vi "Digital_Bridge_3_kart.vi"() -> ()   [LabVIEW 2014] (continued)
                n1468 = call "Kontrol X.vi"("denge degeri"=1.0, "İterasyon Denge"=w4397, "Denge Kosulu x1_x2"=w4399, "Manuel/Otomatik"=w4405, "frekans index"=w4398) -> ("Denge Seçimi"=w4402:u8, "New İterasyon Denge"=w4401:dbl, "Iterasyon Count Successful"=w4400:dbl, "Start Denge X"=w4403:bool)  [unwired: 7 in]
                n1469 = case shown="True" w4403 {
                  tunnel: w4402 -> [w4413 _]
                  tunnel: w4401 -> [_ _]
                  tunnel: w4400 -> [w4412 _]
                  frame False {
                    n1470 = local write "Iterasyon Successful"(w4412) -> ()
                    n1471 = local write "Denge Seçimi"(w4413) -> ()
                    n1472 = local read "iterasyon AD"() -> (w4407:dbl)
                    n1473 = local write "wagner switch"(TRUE ("10R switch")) -> ()
                    n1474 = local write "count meas"(u16 0 ("count meas")) -> ()
                    n1475 = local write "KONTROL X"(FALSE ("KONTROL X")) -> ()
                    n1476 = local write "Boolean"(TRUE ("Boolean 4")) -> ()
                    n1477 = Increment(x=w4407) -> (x+1=w4406:dbl)
                    n1478 = local write "iterasyon AD"(w4406) -> ()
                  }
                  frame True {
                    n1479 = local write "RESET SENS X"(TRUE ("Start Wagner Y")) -> ()
                    n1480 = local write "KONTROL X"(FALSE ("KONTROL X")) -> ()
                  }
                }
              }
            }
            n1481 = case shown="True" "KONTROL Y" {
              frame False {
              }
              frame True {
                n1482 = local read "Outpu Denge Kosulu y1_y2"() -> (w4479:dbl[][])
                n1483 = local read "iterasyon AD"() -> (w4477:dbl)
                n1484 = local read "Manuel/Otomatik"() -> (w4485:enum16{"Manuel", "Otomatik"})
                n1485 = local read "frekans index"() -> (w4478:dbl)
                n1486 = call "Kontrol Y.vi"("denge degeri"=1.0, "İterasyon Denge"=w4477, "Denge Kosulu y1_y2"=w4479, "Manuel/Otomatik"=w4485, "frekans index"=w4478) -> ("Denge Seçimi"=w4482:u8, "New İterasyon Denge"=w4481:dbl, "Iterasyon Count Successful"=w4480:dbl, "Start Denge Y"=w4483:bool)  [unwired: 7 in]
                n1487 = case shown="True" w4483 {
                  tunnel: w4482 -> [w4493 _]
                  tunnel: w4481 -> [_ _]
                  tunnel: w4480 -> [w4492 _]
                  frame False {
                    n1488 = local write "Iterasyon Successful"(w4492) -> ()
                    n1489 = local write "wagner switch"(TRUE ("10R switch")) -> ()
                    n1490 = local write "Denge Seçimi"(w4493) -> ()
                    n1491 = local write "count meas"(u16 0 ("count meas")) -> ()
                    n1492 = local read "iterasyon AD"() -> (w4487:dbl)
                    n1493 = local write "KONTROL Y"(FALSE ("KONTROL Y")) -> ()
                    n1494 = local write "Boolean"(TRUE ("Boolean 4")) -> ()
                    n1495 = Increment(x=w4487) -> (x+1=w4486:dbl)
                    n1496 = local write "iterasyon AD"(w4486) -> ()
                  }
                  frame True {
                    n1497 = local write "RESET SENS Y"(TRUE ("Start Wagner Y")) -> ()
                    n1498 = local write "KONTROL Y"(FALSE ("KONTROL Y")) -> ()
                  }
                }
              }
            }
          }
          frame 2 {
            # "Bu bölümde, ilgili denge durumunun dengede olup olmadığı kontrol edilir.\n\nEğer denge sağlanmışsa, program doğrudan bir sonraki denge aşamasına geçer.\n\nAyrıca, tüm dengeler başarıyla tamamlanmış ve belirlenen ölçüm sayısına ulaşılmışsa, veriler bu alt program (subVI) aracılığıyla Excel dosyasına aktarılır."
            # "Bu bölümde, Y değerinin dengelendiği kabul edilerek, şimdi sıra X değerinin dengede olup olmadığını kontrol etmeye gelir. \n\nEğer X de dengedeyse, program bir sonraki işlem için ilgili switch case’i aktif eder. \n\nAncak Y dengede değilse, program X’i dengelemeye yönelik işlemlere yönlendirilir."
            # "Bu bölümde, X değerinin dengelendiği kabul edilerek, şimdi sıra Y değerinin dengede olup olmadığını kontrol etmeye gelir. \n\nEğer Y de dengedeyse, program bir sonraki işlem için ilgili switch case’i aktif eder. \n\nAncak Y dengede değilse, program Y’yi dengelemeye yönelik işlemlere yönlendirilir."
            # "Bu bölümde ilk olarak giriş (input) değeri sisteme uygulanır. Eğer program ilk kez çalıştırılıyorsa, global input üzerinden belirlenen ilk değer (genellikle 0 V) kullanılır. \n\nArdından, cihazdan X değerleri okunur. Bu işlem 10 kez tekrarlanır ve elde edilen ölçümlerin ortalaması alınarak bir sonuç değeri elde edilir. Bu ortalama değer, daha sonra yapılacak işlemlerde kullanılmak üzere saklanır. Özellikle, formül içinde X değerini sıfırlamak için bu bilgiye ihtiyaç duyulur. \n\nEğer girilen input değeri 8 V’tan büyükse, bu durum sistem için güvenli olmayabileceğinden program hata (error) verir ve işlemi durdurur."
            # "Bu bölümün temel amacı, ölçüm aralığını (range) artırmaktır. Program, cihazdan gelen X ve Y değerlerini okuyarak bu değerlerin belirlenen aralık içinde olup olmadığını kontrol eder. \n\nEğer değerler aralık dışındaysa, aralık tekrar artırılır ve ölçüm yeniden yapılır. \n\nAyrıca, bu süreçte input ve output değerleri global değişkenlere kaydedilir. Çünkü sonraki turda, bu kaydedilen değerler farklı bir ölçüm aralığında eğim hesaplaması için kullanılacaktır."
            # "Bu bölümde, sıfırlanacak değer cihazdan okunur. Eğer okunan değer denge koşulunu sağlıyorsa, program Kontrol Y Case’ine geçer. \n\nAncak denge koşulu sağlanmazsa, program if-else yapısına yönlendirilir ve buna göre işlem devam eder."
            # "Bu bölümde, cihaza ikinci input değeri uygulanır ve karşılık gelen output değeri okunur. Daha sonra, hem input hem de output değerleri bir formüle yerleştirilir. Bu formül sayesinde, cihazın 0’a eşitleyeceği (sıfırlayacağı) yeni bir input değeri hesaplanır ve bu değer cihaza uygulanır."
            # "Auto Phase, Read X1 Y1, Read X2 Y2, Result Phase: \n\nBu bölümler genel olarak faz ölçümü işlemini gerçekleştirir. \n\nİlk olarak, faz değeri 0’a sıfırlanır. Ardından, global input üzerinden belirlenen range (ölçüm aralığı) değeri uygulanır. Bu işlemden sonra yine global input’ta tanımlanmış olan: \n\nInput 1 verilir ve okuma yapılır (Read X1 Y1) \n\nInput 2 verilir ve okuma yapılır (Read X2 Y2) \n\nBu iki ölçüm sonucuna göre faz değeri bir formül yardımıyla hesaplanır. Elde edilen bu yeni faz değeri, ilgili F/P (frekans/faz) dizisine aktarılır. \n\nBu işlemler, sistemin doğru fazla çalışmasını sağlamak ve sonraki işlemlerde bu bilgiyi referans olarak kullanmak için gerçekleştirilir."
            # "X1 2 ile benzer görevi üstleniyor sadece değerler Y oluyor"
            # "IF ELSE X 2 ile benzer görevi üstleniyor sadece değerler Y oluyor"
            # "X 2 ile benzer görevi üstleniyor sadece değerler Y oluyor"
            # "Range Kontrol X 2 ile benzer görevi üstleniyor sadece değerler Y oluyor"
            # "Bu bölümde, daha önce iterasyon (tekrarlama) yapılıp yapılmadığına bakılarak, programın hangi yöne devam edeceğine karar verilir. \n\nEğer gerekli ise, range kontrolü (ölçüm aralığının uygunluğu) yapılır veya sensitivity ayarlama (cihazın duyarlılığını belirleme) bölümlerine yönlendirilir. Bu sayede sistem, ölçüm koşullarına en uygun şekilde ayarlanarak doğru ve güvenilir sonuçlar elde edilmesi sağlanır."
            # "Bu bölümde, daha önce belirlenen F/P dizilerindeki (frekans/faz değerleri) faz bilgileri, mevcut frekansa göre uygulanır. Ardından, ilgili denge koşulunun daha önce gerçekleştirilip gerçekleştirilmediği kontrol edilir. \nEğer bu denge daha önce sağlanmamışsa, program uygun faz ayarlamasını yapar. Ancak denge daha önce zaten kurulmuşsa, faz ayarı yapılmadan işleme devam edilir. Bu sayede gereksiz tekrarların önüne geçilmiş olur."
            # "Bu bölüm, iterasyona (tekrarlamalı işleme) bağlı olarak Reserve ayarının maksimumda mı yoksa minimumda mı olacağını belirler. Aynı zamanda, ölçüm sürecinin başlangıcında kullanılacak olan sensitivity  değerleri de bu bölümde ayarlanır. Bu ayarlar, ölçüm sırasında cihazın hassasiyetini ve çalışma aralığını doğru şekilde belirlemek için gereklidir."
            # "Bu bölümde öncelikle, sistemin kaç kez ölçüm yaptığına işaret eden meas number (ölçüm sayısı) kontrol edilir. \nEğer bu sayı 6’dan büyükse (bu sınır kullanıcı tarafından belirlenmiştir ve değiştirilebilir), program hata verir ve reset values adlı bölüme yönlenir. Bu durum, sistemin çok fazla başarısız deneme yapmasını engellemek içindir. \nEğer ölçüm sayısı 6’dan küçükse, program global bir değişken olan sensitivity (duyarlılık) değerini ayarlar ve ardından işlemlere devam etmek üzere Start X bölümüne geçer."
            # "Bu bölümde, ölçüm için gerekli olan giriş (input) değerleri sisteme girilir. Girişler tamamlandıktan sonra program, ölçüm işlemini başlatmak üzere X adlı bölüme yönlendirilir. Bu adım, ölçüm sürecinin fiilen başlatıldığı ilk noktadır."
            # "Pass subvi girmeden önce doğru range miyiz değil miyiz ölçüyor, değil ise +2 üst kademeye gidiyor"
            # "Start 10R X ile benzer görevi üstleniyor sadece değerler Y oluyor"
            # "Reset Sens X 2 ile benzer görevi üstleniyor sadece değerler Y oluyor"
            # "Start X 2 ile benzer görevi üstleniyor sadece değerler Y oluyor"
            # "10R"
            n1499 = case shown="True" "Start 10R Y" {
              frame False {
              }
              frame True {
                n1500 = flat-sequence {
                  tunnel: [w5317] -> w5305
                  tunnel: [w5316] -> w5304
                  tunnel: w5305 -> [w5321]
                  tunnel: w5304 -> [w5320]
                  frame #0 {
                    n1501 = local read "frekans index"() -> (w5311:dbl)
                    n1502 = local read "Frekanslar"() -> (w5312:dbl[])
                    n1503 = local read "Direnc 1 - Direnc 2"() -> (w5314:u32)
                    n1504 = local read "10R F/P Array"() -> (w5315:dbl[][])
                    n1505 = Index Array(array=w5312, index=w5311) -> (element=w5313:dbl)
                    n1506 = call "get_phase_element.vi"("index r"=w5314, "hz"=w5313, "Array"=w5315) -> ("element"=w5307:dbl)  [unwired: 8 in]
                    n1507 = Number To Fractional String(number=w5307) -> (F-format string=w5308:string)  [unwired: 3 in]
                    n1508 = Search and Replace String(input string=w5308, search string=",", replace string="." ("replace string (\"\")")) -> (result string=w5306:string)  [unwired: 5 in, 3 out]
                    n1509 = local read "GPIB In"() -> (w5318:refnum<visa-resource-name>)
                    n1510 = call "reference phase.vi"("Reference Phase (0.000 degrees)"=w5306, "VISA resource name"=w5318) -> ("error out"=w5316:errorcluster, "VISA resource name out"=w5317:refnum<visa-resource-name>)  [unwired: 8 in]
                  }
                  frame #1 {
                    w5319 = u16 0 items=["A", "A-B"] ("Input Source (0: A)")
                    n1511 = call "input source.vi"("error in (no error)"=w5320, "Input Source (0: A)"=w5319, "VISA resource name"=w5321) -> ()  [unwired: 7 in, 2 out]
                  }
                  frame #2 {
                    n1512 = local write "Boolean 2"(FALSE ("Boolean 4")) -> ()
                    n1513 = local write "RESET SENS Y 2"(TRUE ("START X")) -> ()
                    n1514 = local write "Start 10R Y"(FALSE ("START Y 6")) -> ()
                  }
                }
              }
            }
            n1515 = case shown="True" "10R switch" {
              frame False {
              }
              frame True {
                n1516 = flat-sequence {
                  frame #0 {
                    n1517 = local read "iterasyon 10R"() -> (w5245:dbl)
                    n1518 = Equal?(x=w5245, y=0.0) -> (x = y?=w5246:bool)
                    n1519 = case shown="True" w5246 {
                      frame False {
                      }
                      frame True {
                        n1520 = local read "1 or 10"() -> (w5248:i32)
                        n1521 = case shown="1" w5248 {
                          frame 0, Default {
                          }
                          frame 1 {
                            n1522 = local write "iterasyon 10R"(1.0 ("iterasyon WAGNER")) -> ()
                          }
                        }
                      }
                    }
                  }
                  frame #1 {
                    n1523 = local read "iterasyon 10R"() -> (w5251:dbl)
                    n1524 = Greater?(x=w5251, y=0.0) -> (0:w5250:bool)
                    n1525 = case shown="True" w5250 {
                      frame False {
                        n1526 = local read "Reserve 10R"() -> (w5254:u16)
                        n1527 = case shown="2" w5254 {
                          tunnel: ["0" ("Reserve(MAX-MIN)") "1" ("Reserve(MAX-MIN)") "2" ("Reserve(MAX-MIN)")] -> w5253
                          frame 0, Default {
                          }
                          frame 1 {
                          }
                          frame 2 {
                          }
                        }
                        n1528 = local read "GPIB In"() -> (w5255:refnum<visa-resource-name>)
                        n1529 = call "Reserve.vi"("Reserve(MAX-MIN)"=w5253, "VISA resource name"=w5255) -> ()  [unwired: 8 in, 2 out]
                      }
                      frame True {
                        n1530 = local read "GPIB In"() -> (w5260:refnum<visa-resource-name>)
                        n1531 = call "Reserve.vi"("Reserve(MAX-MIN)"="0", "VISA resource name"=w5260) -> ()  [unwired: 8 in, 2 out]
                      }
                    }
                  }
                  frame #2 {
                    n1532 = Wait (ms)(milliseconds to wait=u32 500) -> ()  [unwired: 1 out]
                  }
                  frame #3 {
                    w5263 = u16 1 items=["Wagner", "Ground"] ("Switch")
                    w5264 = u16 2 items=["Open All", "Ana Denge", "10R", "1R"] ("Ring")
                    n1533 = call "mux1.vi"("Ring"=w5264) -> ("error out"=w5265:errorcluster)  [unwired: 9 in]
                    n1534 = property on="Tab Control" class="TabCtl (strict)"("Value"=T4."10R" ("Tab Control")) -> ()  [unwired: 2 in, 2 out]
                    n1535 = call "mux2.vi"("Switch"=w5263, "error in (no error)"=w5265) -> ()  [unwired: 6 in, 1 out]
                  }
                  frame #4 {
                    n1536 = Wait (ms)(milliseconds to wait=u32 1000) -> ()  [unwired: 1 out]
                  }
                  frame #5 {
                    n1537 = local read "1 or 10"() -> (w5270:i32)
                    n1538 = local read "İterasyon X 2"() -> (w5273:dbl)
                    n1539 = Equal?(x=w5270, y=1) -> (x = y?=w5269:bool)
                    n1540 = Greater?(x=w5273, y=0.0) -> (0:w5268:bool)
                    n1541 = Or(x=w5268, y=w5269) -> (x .or. y?=w5267:bool)
                    n1542 = case shown="False" w5267 {
                      frame False {
                        n1543 = local read "X Range 10R"() -> (w5275:dbl)
                        n1544 = local read "Y Range 10R"() -> (w5274:dbl)
                        n1545 = global write "show_sensitivity.vi" "show sensitivity (10R  x)"(w5275) -> ()
                        n1546 = global write "show_sensitivity.vi" "show sensitivity (10R  y)"(w5274) -> ()
                      }
                      frame True {
                        w5276 = 16.0 ("Max. Hassasiyet")
                        n1547 = global write "show_sensitivity.vi" "show sensitivity (10R  x)"(w5276) -> ()
                        n1548 = global write "show_sensitivity.vi" "show sensitivity (10R  y)"(w5276) -> ()
                      }
                    }
                  }
                  frame #6 {
                    n1549 = local write "Start 10R X"(TRUE ("START WAGNER")) -> ()
                    n1550 = local write "10R switch"(FALSE ("wagner switch")) -> ()
                  }
                }
              }
            }
            n1551 = case shown="True" "RESET SENS Y 2" {
              frame False {
              }
              frame True {
                n1552 = local read "count meas"() -> (w5284:u16)
                n1553 = local read "iterasyon 10R"() -> (w5282:dbl)
                n1554 = Greater?(x=w5284, y=u16 8) -> (0:w5281:bool)
                n1555 = Greater?(x=w5282, y=10.0) -> (0:w5280:bool)
                n1556 = Or(x=w5281, y=w5280) -> (x .or. y?=w5279:bool)
                n1557 = case shown="True" w5279 {
                  frame False {
                    n1558 = flat-sequence {
                      frame #0 {
                        n1559 = global read "show_sensitivity.vi" "show sensitivity (10R  y)"() -> (w5286:dbl)
                        n1560 = local read "GPIB In"() -> (w5287:refnum<visa-resource-name>)
                        n1561 = call "get_sensitivity.vi"("input 1"=w5286, "SR850 GPIB In"=w5287) -> ()  [unwired: 8 in, 2 out]
                      }
                      frame #1 {
                        n1562 = Wait (ms)(milliseconds to wait=u32 500) -> ()  [unwired: 1 out]
                      }
                      frame #2 {
                        n1563 = local write "RESET SENS Y 2"(FALSE ("RESET SENS X")) -> ()
                        n1564 = local write "START Y 2"(TRUE ("START X 4")) -> ()
                      }
                    }
                  }
                  frame True {
                    n1565 = local read "iterasyon 10R"() -> (w5293:dbl)
                    n1566 = Greater?(x=w5293, y=10.0) -> (0:w5291:bool)
                    n1567 = case shown="False" w5291 {
                      frame False {
                        n1568 = flat-sequence {
                          frame #0 {
                            n1569 = local write "count meas"(u16 9 ("count meas")) -> ()
                            n1570 = local write "RESET SENS Y 2"(FALSE ("Start 10R X")) -> ()
                            n1571 = local write "İterasyon X 2"(0.0 ("İterasyon X 2")) -> ()
                          }
                          frame #1 {
                            n1572 = local write "reset values"(TRUE ("Start 10R X")) -> ()
                            n1573 = local write "error"(TRUE ("Start 10R X")) -> ()
                          }
                        }
                      }
                      frame True {
                        n1574 = flat-sequence {
                          frame #0 {
                            n1575 = local write "count meas"(u16 10 ("count meas")) -> ()
                            n1576 = local write "RESET SENS Y 2"(FALSE ("Start 10R X")) -> ()
                            n1577 = local write "İterasyon X 2"(0.0 ("İterasyon X 2")) -> ()
                          }
                          frame #1 {
                            n1578 = local write "reset values"(TRUE ("Start 10R X")) -> ()
                            n1579 = local write "error"(TRUE ("Start 10R X")) -> ()
                          }
                        }
                      }
                    }
                  }
                }
              }
            }
            n1580 = case shown="True" "RESET SENS X 2" {
              frame False {
              }
              frame True {
                n1581 = local read "iterasyon 10R"() -> (w5333:dbl)
                n1582 = local read "count meas"() -> (w5335:u16)
                n1583 = Greater?(x=w5335, y=u16 8) -> (0:w5331:bool)
                n1584 = Greater?(x=w5333, y=5.0) -> (0:w5332:bool)
                n1585 = Or(x=w5331, y=w5332) -> (x .or. y?=w5330:bool)
                n1586 = case shown="True" w5330 {
                  frame False {
                    n1587 = flat-sequence {
                      frame #0 {
                        n1588 = global read "show_sensitivity.vi" "show sensitivity (10R  x)"() -> (w5337:dbl)
                        n1589 = local read "GPIB In"() -> (w5338:refnum<visa-resource-name>)
                        n1590 = call "get_sensitivity.vi"("input 1"=w5337, "SR850 GPIB In"=w5338) -> ()  [unwired: 8 in, 2 out]
                      }
                      frame #1 {
                        n1591 = Wait (ms)(milliseconds to wait=u32 500) -> ()  [unwired: 1 out]
                      }
                      frame #2 {
                        n1592 = local write "RESET SENS X 2"(FALSE ("RESET SENS X")) -> ()
                        n1593 = local write "START X 2"(TRUE ("START X 4")) -> ()
                      }
                    }
                  }
                  frame True {
                    n1594 = local read "iterasyon 10R"() -> (w5344:dbl)
                    n1595 = Greater?(x=w5344, y=5.0) -> (0:w5342:bool)
                    n1596 = case shown="False" w5342 {
                      frame False {
                        n1597 = flat-sequence {
                          frame #0 {
                            n1598 = local write "İterasyon X 2"(0.0 ("İterasyon X 2")) -> ()
                            n1599 = local write "count meas"(u16 9 ("count meas")) -> ()
                            n1600 = local write "RESET SENS X 2"(FALSE ("Start 10R X")) -> ()
                          }
                          frame #1 {
                            n1601 = local write "reset values"(TRUE ("Start 10R X")) -> ()
                            n1602 = local write "error"(TRUE ("Start 10R X")) -> ()
                          }
                        }
                      }
                      frame True {
                        n1603 = flat-sequence {
                          frame #0 {
                            n1604 = local write "İterasyon X 2"(0.0 ("İterasyon X 2")) -> ()
                            n1605 = local write "count meas"(u16 10 ("count meas")) -> ()
                            n1606 = local write "RESET SENS X 2"(FALSE ("Start 10R X")) -> ()
                          }
                          frame #1 {
                            n1607 = local write "reset values"(TRUE ("Start 10R X")) -> ()
                            n1608 = local write "error"(TRUE ("Start 10R X")) -> ()
                          }
                        }
                      }
                    }
                  }
                }
              }
            }
            n1609 = case shown="True" "Start 10R X" {
              frame False {
              }
              frame True {
                n1610 = flat-sequence {
                  frame #0 {
                    w5222 = u16 0 items=["A", "A-B"] ("Input Source (0: A)")
                    n1611 = local read "frekans index"() -> (w5217:dbl)
                    n1612 = local read "Frekanslar"() -> (w5218:dbl[])
                    n1613 = local read "Direnc 1 - Direnc 2"() -> (w5219:u32)
                    n1614 = local read "10R F/P Array"() -> (w5220:dbl[][])
                    n1615 = Index Array(array=w5218, index=w5217) -> (element=w5216:dbl)
                    n1616 = call "get_phase_element.vi"("index r"=w5219, "hz"=w5216, "Array"=w5220) -> ("element"=w5212:dbl)  [unwired: 8 in]
                    n1617 = Number To Fractional String(number=w5212) -> (F-format string=w5215:string)  [unwired: 3 in]
                    n1618 = local read "GPIB In"() -> (w5221:refnum<visa-resource-name>)
                    n1619 = Search and Replace String(input string=w5215, search string=",", replace string="." ("replace string (\"\")")) -> (result string=w5211:string)  [unwired: 5 in, 3 out]
                    n1620 = call "reference phase.vi"("Reference Phase (0.000 degrees)"=w5211, "VISA resource name"=w5221) -> ("error out"=w5223:errorcluster, "VISA resource name out"=w5224:refnum<visa-resource-name>)  [unwired: 8 in]
                    n1621 = call "input source.vi"("error in (no error)"=w5223, "Input Source (0: A)"=w5222, "VISA resource name"=w5224) -> ()  [unwired: 7 in, 2 out]
                  }
                  frame #1 {
                    n1622 = local read "İterasyon X 2"() -> (w5235:dbl)
                    n1623 = local read "frekans index"() -> (w5228:dbl)
                    n1624 = local read "1 or 10"() -> (w5239:i32)
                    n1625 = local read "control hz array"() -> (w5232:dbl[][])
                    n1626 = Greater?(x=w5235, y=0.0) -> (0:w5236:bool)
                    n1627 = call "change2d.vi"("reset(default false)"=FALSE, "index (col)"=w5228, "index (row)"=2, "read/write(T/F)"=TRUE, "2D Array"=w5232) -> ("result count"=w5233:dbl)  [unwired: 5 in, 1 out]
                    n1628 = Equal?(x=w5239, y=1) -> (x = y?=w5237:bool)
                    n1629 = local read "set"() -> (w5234:u16)
                    n1630 = Or(x=w5236, y=w5237) -> (x .or. y?=w5226:bool)
                    n1631 = Equal?(x=w5233, y=w5234) -> (x = y?=w5227:bool)
                    n1632 = Or(x=w5226, y=w5227) -> (x .or. y?=w5225:bool)
                    n1633 = case shown="True" w5225 {
                      frame False {
                        n1634 = local write "auto phase 10R"(TRUE ("auto phase 10R")) -> ()
                        n1635 = local write "Start 10R X"(FALSE ("auto phase 10R")) -> ()
                      }
                      frame True {
                        n1636 = local write "Contiune 10R"(TRUE) -> ()
                        n1637 = local write "Start 10R X"(FALSE ("START WAGNER")) -> ()
                      }
                    }
                  }
                }
              }
            }
            n1638 = case shown="True" "START Y 2" {
              frame False {
              }
              frame True {
                n1639 = flat-sequence {
                  frame #0 {
                    n1640 = local read "10R Y(k-1)"() -> (w5326:dbl)
                    n1641 = local read "10R Yk"() -> (w5325:dbl)
                    n1642 = local write "input 1 y [10R]"(w5325) -> ()
                    n1643 = local write "input 2 y [10R]"(w5326) -> ()
                    n1644 = global write "DB_Global_4_kart-Test.vi" "phase 3/0"(w5325) -> ()
                  }
                  frame #1 {
                    n1645 = Wait (ms)(milliseconds to wait=u32 500) -> ()  [unwired: 1 out]
                  }
                  frame #2 {
                    n1646 = local write "START Y 2"(FALSE ("START X")) -> ()
                    n1647 = local write "Y 2"(TRUE ("START X")) -> ()
                  }
                }
              }
            }
            n1648 = case shown="True" "START X 2" {
              frame False {
              }
              frame True {
                n1649 = flat-sequence {
                  frame #0 {
                    n1650 = local read "10R X(k-1)"() -> (w5356:dbl)
                    n1651 = local read "10R Xk"() -> (w5355:dbl)
                    n1652 = global write "DB_Global_4_kart-Test.vi" "amplitude 3/0"(w5355) -> ()
                    n1653 = local write "input 1 x [10R]"(w5355) -> ()
                    n1654 = local write "input 2 x [10R]"(w5356) -> ()
                  }
                  frame #1 {
                    n1655 = Wait (ms)(milliseconds to wait=u32 500) -> ()  [unwired: 1 out]
                  }
                  frame #2 {
                    n1656 = local write "START X 2"(FALSE ("START X 4")) -> ()
                    n1657 = local write "X 2"(TRUE ("START X")) -> ()
                  }
                  frame #3 {
                  }
                }
              }
            }
            n1658 = case shown="True" "Optimum Range 2" {
              frame False {
              }
              frame True {
                n1659 = flat-sequence {
                  frame #0 {
                    n1660 = global read "show_sensitivity.vi" "show sensitivity (10R  x)"() -> (w4860:dbl)
                    n1661 = local read "GPIB In"() -> (w4859:refnum<visa-resource-name>)
                    n1662 = call "get_sensitivity.vi"("input 1"=w4860, "SR850 GPIB In"=w4859) -> ()  [unwired: 8 in, 2 out]
                  }
                  frame #1 {
                    n1663 = call "set optimum range.vi"("denge degeri"=2.0) -> ("ok"=w4861:bool)  [unwired: 14 in]
                    n1664 = case shown="True" w4861 {
                      frame False {
                      }
                      frame True {
                        n1665 = local write "Optimum Range 2"(FALSE ("Optimum Range 1")) -> ()
                        n1666 = local write "PASS 10R"(TRUE ("PASS 10R")) -> ()
                      }
                    }
                  }
                }
              }
            }
            n1667 = case shown="True" "PASS 10R" {
              frame False {
              }
              frame True {
                n1668 = flat-sequence {
                  tunnel: [w5117] -> w5107
                  tunnel: [w5116] -> w5106
                  tunnel: [w5115] -> w5105
                  tunnel: [w5114] -> w5104
                  tunnel: [w5113] -> w5103
                  tunnel: [w5112] -> w5102
                  tunnel: [w5111] -> w5101
                  tunnel: w5107 -> [w5179]
                  tunnel: w5106 -> [w5178]
                  tunnel: w5105 -> [w5177]
                  tunnel: w5104 -> [w5176]
                  tunnel: w5103 -> [w5175]
                  tunnel: w5102 -> [w5174]
                  tunnel: w5101 -> [w5173]
                  frame #0 {
                    n1669 = Wait (ms)(milliseconds to wait=u32 500) -> ()  [unwired: 1 out]
                  }
                  frame #1 {
                    n1670 = local read "Other Array"() -> (w5145:dbl[])
                    n1671 = for {
                      N: 7 -> [_]
                      shift-right: [w5162] -> w5148
                      shift-left: w5145 -> [w5165]
                      i -> [w5164]
                      n1672 = case shown="6" w5164 {
                        tunnel: [2.0 ("iterasyon WAGNER") w5167 w5168 w5169 w5170 w5171 w5172] -> w5163
                        frame 0, Default {
                        }
                        frame 1 {
                          n1673 = local read "Iterasyon Successful"() -> (w5167:dbl)
                        }
                        frame 2 {
                          n1674 = local read "Direnc 1 - Direnc 2"() -> (w5168:u32)
                        }
                        frame 3 {
                          n1675 = local read "olcum"() -> (w5169:u16)
                        }
                        frame 4 {
                          n1676 = local read "set"() -> (w5170:u16)
                        }
                        frame 5 {
                          n1677 = local read "frekans index"() -> (w5171:dbl)
                        }
                        frame 6 {
                          n1678 = local read "iterasyon 10R"() -> (w5172:dbl)
                        }
                      }
                      n1679 = Replace Array Subset(array=w5165, new element=w5163, index=w5164) -> (w5162:dbl[])
                    }
                    n1680 = control-ref of="Default Values Listbox"() -> (w5135:refnum<vi>)
                    n1681 = local read "Output Denge Kosulu x2_y2"() -> (w5150:dbl[][])
                    n1682 = local read "Output Denge Kosulu x1_x2"() -> (w5131:dbl[][])
                    n1683 = local read "Outpu Denge Kosulu y1_y2"() -> (w5130:dbl[][])
                    n1684 = local read "Frekanslar"() -> (w5110:dbl[])
                    n1685 = local read "Cluster"() -> (w5133:T2)
                    n1686 = local read "Cluster 2"() -> (w5132:T1)
                    n1687 = Array Size(array=w5110) -> (size(s)=w5109:i32)
                    n1688 = local read "input values"() -> (w5134:dbl[])
                    n1689 = local read "default values"() -> (w5149:T3)
                    n1690 = call "merge_x_y.vi"("frekans size"=w5109, "y1_y2"=w5130, "x1_x2"=w5131) -> ("x1_x2_y1_y2"=w5129:dbl[][])  [unwired: 8 in]
                    n1691 = local read "Sheet name"() -> (w5146:string)
                    n1692 = local read "Other Boolean Array"() -> (w5144:bool[])
                    n1693 = for {
                      N: 5 -> [_]
                      shift-right: [w5153] -> w5147
                      shift-left: w5144 -> [w5156]
                      i -> [w5155]
                      n1694 = case shown="1" w5155 {
                        tunnel: [FALSE FALSE FALSE FALSE FALSE] -> w5154
                        frame 0, Default {
                        }
                        frame 1 {
                        }
                        frame 2 {
                        }
                        frame 3 {
                        }
                        frame 4 {
                        }
                      }
                      n1695 = Replace Array Subset(array=w5156, new element=w5154, index=w5155) -> (w5153:bool[])
                    }
                    n1696 = call "Pass.vi"("Other Array"=w5148, "Other Boolean Array"=w5147, "Denge Kosulu x2_y2"=w5150, "LstBox Refnum"=w5135, "Cluster"=w5133, "F/P Array Cluster"=w5132, "Sheet name"=w5146, "default values"=w5149, "x1_x2_y1_y2"=w5129, "input values"=w5134) -> ("output values"=w5128:dbl[], "Output Other Boolean Array"=w5141:bool[], "Output Cluster"=w5127:T2, "Output F/P Array Cluster"=w5123:T1, "output default values"=w5143:T11, "Output Iterasyon Successful"=w5142:dbl, "Denge Seçimi"=w5115:u8, "end time"=w5113:string)  [unwired: 1 in, 1 out]
                    n1697 = Unbundle By Name(w5127) -> ("F Values Array"=w5126:dbl[][], "control hz array"=w5125:dbl[][], "extra default values"=w5124:dbl[][])
                    n1698 = local write "input values"(w5128) -> ()
                    n1699 = Unbundle By Name(w5123) -> ("AD F/P Array"=w5122:dbl[][], "10R F/P Array"=w5121:dbl[][], "1R F/P Array"=w5120:dbl[][], "Wagner F/P Array"=w5119:dbl[][], "Kelvin F/P Array"=w5118:dbl[][])
                    n1700 = local write "default values"(w5143) -> ()
                    n1701 = local write "Iterasyon Successful"(w5142) -> ()
                    n1702 = local write "AD F/P Array"(w5122) -> ()
                    n1703 = local write "10R F/P Array"(w5121) -> ()
                    n1704 = local write "1R F/P Array"(w5120) -> ()
                    n1705 = local write "Wagner F/P Array"(w5119) -> ()
                    n1706 = local write "Kelvin F/P Array"(w5118) -> ()
                    n1707 = local write "F Values Array"(w5126) -> ()
                    n1708 = local write "control hz array"(w5125) -> ()
                    n1709 = local write "extra default values"(w5124) -> ()
                    n1710 = Index Array(array=w5141, index #1=0 ("index"), index #2=1 ("index"), index #3=2 ("index"), index #4=3 ("index"), index #5=4 ("index")) -> (element #1=w5117:bool, element #2=w5116:bool, element #3=w5114:bool, element #4=w5112:bool, element #5=w5111:bool)
                  }
                  frame #2 {
                    n1711 = case shown="True" w5179 {
                      frame False {
                      }
                      frame True {
                        n1712 = local write "reset values"(TRUE ("reset values")) -> ()
                        n1713 = local write "Boolean 2"(TRUE ("Boolean 4")) -> ()
                        n1714 = local write "pass hz"(TRUE ("pass hz")) -> ()
                        n1715 = local write "PASS 10R"(FALSE ("PASS 10R")) -> ()
                      }
                    }
                    n1716 = case shown="True" w5178 {
                      tunnel: w5177 -> [_ w5195]
                      frame False {
                      }
                      frame True {
                        n1717 = local write "1R switch"(TRUE ("10R switch")) -> ()
                        n1718 = local write "count meas"(u16 0 ("count meas")) -> ()
                        n1719 = local write "Denge Seçimi"(w5195) -> ()
                        n1720 = local write "Boolean 2"(TRUE ("Boolean 4")) -> ()
                        n1721 = local write "PASS 10R"(FALSE ("PASS 10R")) -> ()
                        n1722 = local read "cycle 10r 1r"() -> (w5189:bool[])
                        n1723 = Replace Array Subset(array=w5189, new element=TRUE ("new element/subarray"), index=0) -> (w5190:bool[])
                        n1724 = local write "cycle 10r 1r"(w5190) -> ()
                      }
                    }
                    n1725 = case shown="True" w5173 {
                      frame False {
                      }
                      frame True {
                        n1726 = local write "RESET SENS Y 2"(TRUE ("RESET SENS Y 4")) -> ()
                        n1727 = local write "PASS 10R"(FALSE ("PASS 10R")) -> ()
                      }
                    }
                    n1728 = case shown="True" w5174 {
                      frame False {
                      }
                      frame True {
                        n1729 = local write "RESET SENS X 2"(TRUE ("RESET SENS X 4")) -> ()
                        n1730 = local write "PASS 10R"(FALSE ("PASS 10R")) -> ()
                      }
                    }
                    n1731 = case shown="True" w5176 {
                      tunnel: w5175 -> [_ w5186]
                      frame False {
                      }
                      frame True {
                        n1732 = local write "reset values"(TRUE ("reset values")) -> ()
                        n1733 = local write "end time"(w5186) -> ()
                        n1734 = local write "PASS 10R"(FALSE ("PASS 10R")) -> ()
                        n1735 = local write "Boolean 2"(TRUE ("Boolean 4")) -> ()
                      }
                    }
                  }
                  frame #3 {
                  }
                }
              }
            }
            n1736 = case shown="True" "Contiune 10R" {
              frame False {
              }
              frame True {
                n1737 = local read "iterasyon 10R"() -> (w4919:dbl)
                n1738 = local read "1 or 10"() -> (w4915:i32)
                n1739 = local read "frekans index"() -> (w4914:dbl)
                n1740 = local read "control hz array"() -> (w4910:dbl[][])
                n1741 = call "change2d.vi"("reset(default false)"=FALSE, "index (col)"=w4914, "index (row)"=2, "read/write(T/F)"=TRUE, "2D Array"=w4910) -> ("result count"=w4909:dbl)  [unwired: 5 in, 1 out]
                n1742 = local read "set"() -> (w4908:u16)
                n1743 = case shown="1" w4915 {
                  tunnel: [FALSE TRUE] -> w4916
                  frame 10, Default {
                  }
                  frame 1 {
                  }
                }
                n1744 = Greater?(x=w4919, y=0.0) -> (0:w4917:bool)
                n1745 = Equal?(x=w4909, y=w4908) -> (x = y?=w4907:bool)
                n1746 = Or(x=w4917, y=w4916) -> (x .or. y?=w4906:bool)
                n1747 = Or(x=w4906, y=w4907) -> (x .or. y?=w4905:bool)
                n1748 = case shown="True" w4905 {
                  frame False {
                    n1749 = local write "RESET SENS X 2"(TRUE ("START X")) -> ()
                    n1750 = local write "Contiune 10R"(FALSE ("START WAGNER")) -> ()
                    n1751 = local write "Boolean 2"(FALSE ("Boolean 4")) -> ()
                  }
                  frame True {
                    n1752 = local write "Optimum Range 2"(TRUE ("START X")) -> ()
                    n1753 = local write "Contiune 10R"(FALSE ("Boolean 4")) -> ()
                    n1754 = local write "Boolean 2"(FALSE ("Boolean 4")) -> ()
                  }
                }
              }
            }
            n1755 = case shown="True" "auto phase 10R" {
              frame False {
              }
              frame True {
                n1756 = flat-sequence {
                  frame #0 {
                    n1757 = local read "GPIB In"() -> (w5202:refnum<visa-resource-name>)
                    n1758 = call "reference phase.vi"("Reference Phase (0.000 degrees)"="0", "VISA resource name"=w5202) -> ()  [unwired: 8 in, 2 out]
                  }
                  frame #1 {
                    w5204 = u16 0 items=["100 nV", "200 nV", "500 nV", "1 uV", "2 uV", "5 uV", "10 uV", "20 uV", "50 uV", "100 uV", "200 uV", "500 uV", "1 mV"] ("Min. Hassasiyet")
                    n1759 = local read "GPIB In"() -> (w5205:refnum<visa-resource-name>)
                    n1760 = local read "X Range 10R"() -> (w5203:dbl)
                    n1761 = call "GAIN BASIC.vi"("SR850 GPIB In"=w5205, "Max. Hassasiyet"=w5203, "Auto Gain (False)"=FALSE, "Min. Hassasiyet"=w5204) -> ()  [unwired: 10 in, 2 out]
                  }
                  frame #2 {
                    n1762 = local read "X 1.input 10R"() -> (w5207:dbl)
                    n1763 = global write "DB_Global_4_kart-Test.vi" "amplitude 3/0"(w5207) -> ()
                    n1764 = global write "DB_Global_4_kart-Test.vi" "phase 3/0"(w5207) -> ()
                  }
                  frame #3 {
                    n1765 = Wait (ms)(milliseconds to wait=u32 750) -> ()  [unwired: 1 out]
                  }
                  frame #4 {
                    n1766 = local write "read x1 y1 2"(TRUE ("output x")) -> ()
                    n1767 = local write "auto phase 10R"(FALSE ("auto phase wagner")) -> ()
                  }
                }
              }
            }
            n1768 = case shown="True" "RANGE KONTROL Y 2" {
              frame False {
              }
              frame True {
                n1769 = local read "Outpu Denge Kosulu y1_y2"() -> (w4972:dbl[][])
                n1770 = local read "input 1 y [10R]"() -> (w4973:dbl)
                n1771 = local read "iterasyon 10R"() -> (w4971:dbl)
                n1772 = local read "frekans index"() -> (w4965:dbl)
                n1773 = local read "input 2 y [10R]"() -> (w4974:dbl)
                n1774 = local read "output 2 y [10R]"() -> (w4968:dbl)
                n1775 = local read "output 1 y [10R]"() -> (w4970:dbl)
                n1776 = call "Range Kontrol Y.vi"("denge degeri"=2.0, "iterasyon Denge"=w4971, "frekans index"=w4965, "Denge Kosulu y1_y2"=w4972, "Yk"=w4973, "Y(k-1)"=w4974, "output y 1"=w4970, "output y 2"=w4968) -> ("Output Y(k-1)"=w4964:dbl, "result output y"=w4975:dbl, "KONTROL X"=w4967:bool, "IF ELSE"=w4966:bool)  [unwired: 8 in]
                n1777 = local write "10R Y(k-1)"(w4964) -> ()
                n1778 = local write "result output y [10R]"(w4975) -> ()
                n1779 = flat-sequence {
                  tunnel: w4967 -> [w4977]
                  tunnel: w4966 -> [w4976]
                  frame #0 {
                    n1780 = case shown="True" w4976 {
                      frame False {
                      }
                      frame True {
                        n1781 = local write "IF ELSE Y 2"(TRUE ("IF ELSE X 4")) -> ()
                      }
                    }
                    n1782 = case shown="True" w4977 {
                      frame False {
                      }
                      frame True {
                        n1783 = local write "KONTROL X 2"(TRUE ("KONTROL Y 4")) -> ()
                      }
                    }
                  }
                  frame #1 {
                    n1784 = local write "RANGE KONTROL Y 2"(FALSE ("KONTROL Y 4")) -> ()
                    n1785 = local read "İterasyon Y 2"() -> (w4980:dbl)
                    n1786 = Increment(x=w4980) -> (x+1=w4981:dbl)
                    n1787 = local write "İterasyon Y 2"(w4981) -> ()
                  }
                }
              }
            }
            n1788 = case shown="True" "RANGE KONTROL X 2" {
              frame False {
              }
              frame True {
                n1789 = local read "Output Denge Kosulu x1_x2"() -> (w5058:dbl[][])
                n1790 = local read "input 1 x [10R]"() -> (w5059:dbl)
                n1791 = local read "iterasyon 10R"() -> (w5057:dbl)
                n1792 = local read "frekans index"() -> (w5050:dbl)
                n1793 = local read "input 2 x [10R]"() -> (w5060:dbl)
                n1794 = local read "output 2 x [10R]"() -> (w5054:dbl)
                n1795 = local read "output 1 x [10R]"() -> (w5056:dbl)
                n1796 = call "Range Kontrol X.vi"("denge degeri"=2.0, "iterasyon Denge"=w5057, "frekans index"=w5050, "Denge Kosulu x1_x2"=w5058, "Xk"=w5059, "X(k-1)"=w5060, "output x 1"=w5056, "output x 2"=w5054) -> ("Output X(k-1)"=w5049:dbl, "result output x"=w5061:dbl, "KONTROL Y"=w5053:bool, "IF ELSE"=w5052:bool, "Start Denge Y"=w5051:bool)  [unwired: 7 in]
                n1797 = local write "10R X(k-1)"(w5049) -> ()
                n1798 = local write "result output x [10R]"(w5061) -> ()
                n1799 = flat-sequence {
                  tunnel: w5053 -> [w5064]
                  tunnel: w5052 -> [w5063]
                  tunnel: w5051 -> [w5062]
                  frame #0 {
                    n1800 = case shown="True" w5062 {
                      frame False {
                      }
                      frame True {
                        n1801 = local write "Start 10R Y"(TRUE ("Start Wagner Y")) -> ()
                      }
                    }
                    n1802 = case shown="True" w5063 {
                      frame False {
                      }
                      frame True {
                        n1803 = local write "IF ELSE X 2"(TRUE ("IF ELSE X 4")) -> ()
                      }
                    }
                    n1804 = case shown="True" w5064 {
                      frame False {
                      }
                      frame True {
                        n1805 = local write "KONTROL Y 2"(TRUE ("KONTROL Y 4")) -> ()
                      }
                    }
                  }
                  frame #1 {
                    n1806 = local write "RANGE KONTROL X 2"(FALSE ("KONTROL Y 4")) -> ()
                    n1807 = local read "İterasyon X 2"() -> (w5069:dbl)
                    n1808 = Increment(x=w5069) -> (x+1=w5068:dbl)
                    n1809 = local write "İterasyon X 2"(w5068) -> ()
                  }
                }
              }
            }
            n1810 = case shown="True" "X 2" {
              frame False {
              }
              frame True {
                n1811 = local read "İterasyon X 2"() -> (w5092:dbl)
                n1812 = local read "10R X(k-1)"() -> (w5093:dbl)
                n1813 = call "X.vi"("X(k-1)"=w5093, "İterasyon Denge"=w5092, "denge degeri"=2.0) -> ("error"=w5090:bool, "output X(k-1)"=w5087:dbl, "output x 1"=w5088:dbl, "cycle"=w5089:bool)  [unwired: 5 in]
                n1814 = case shown="False" w5089 {
                  tunnel: w5090 -> [w5096 _]
                  tunnel: w5088 -> [w5095 _]
                  tunnel: w5087 -> [w5094 _]
                  frame False {
                    n1815 = case shown="False" w5096 {
                      frame False {
                        n1816 = local write "X1 2"(TRUE ("X1 4")) -> ()
                        n1817 = local write "X 2"(FALSE ("X 4")) -> ()
                      }
                      frame True {
                        n1818 = local write "X 2"(FALSE ("X 4")) -> ()
                        n1819 = local write "error"(TRUE ("X1 4")) -> ()
                      }
                    }
                    n1820 = local write "output 1 x [10R]"(w5095) -> ()
                    n1821 = local write "input 2 x [10R]"(w5094) -> ()
                    n1822 = local write "10R X(k-1)"(w5094) -> ()
                  }
                  frame True {
                  }
                }
              }
            }
            n1823 = case shown="True" "read x1 y1 2" {
              frame False {
              }
              frame True {
                n1824 = local read "X Range 10R"() -> (w4843:dbl)
                n1825 = call "only_x_and_y_output.vi"("range"=w4843) -> ("cycle 2"=w4847:bool, "range 2"=w4844:dbl, "Output Y"=w4845:dbl, "Output X"=w4846:dbl)  [unwired: 7 in]
                n1826 = case shown="False" w4847 {
                  tunnel: w4846 -> [w4850 _]
                  tunnel: w4845 -> [w4849 _]
                  tunnel: w4844 -> [w4848 w4858]
                  frame False {
                    n1827 = flat-sequence {
                      tunnel: w4850 -> [w4853]
                      tunnel: w4849 -> [w4852]
                      tunnel: w4848 -> [w4851]
                      frame #0 {
                        n1828 = local write "X Range 10R"(w4851) -> ()
                        n1829 = local write "Output Y1"(w4852) -> ()
                        n1830 = local write "Output X1"(w4853) -> ()
                      }
                      frame #1 {
                        n1831 = local read "X 2.input 10R"() -> (w4854:dbl)
                        n1832 = global write "DB_Global_4_kart-Test.vi" "amplitude 3/0"(w4854) -> ()
                      }
                      frame #2 {
                        n1833 = Wait (ms)(milliseconds to wait=u32 750) -> ()  [unwired: 1 out]
                      }
                      frame #3 {
                        n1834 = local write "read x2 y2 2"(TRUE ("output x")) -> ()
                        n1835 = local write "read x1 y1 2"(FALSE ("output x")) -> ()
                      }
                    }
                  }
                  frame True {
                    n1836 = local write "X Range 10R"(w4858) -> ()
                  }
                }
              }
            }
            n1837 = case shown="True" "Y 2" {
              frame False {
              }
              frame True {
                n1838 = local read "İterasyon Y 2"() -> (w5004:dbl)
                n1839 = local read "10R Y(k-1)"() -> (w5005:dbl)
                n1840 = call "Y.vi"("Y(k-1)"=w5005, "İterasyon Denge"=w5004, "denge degeri"=2.0) -> ("error"=w5002:bool, "output Y(k-1)"=w4999:dbl, "output y 1"=w5000:dbl, "cycle"=w5001:bool)  [unwired: 5 in]
                n1841 = case shown="False" w5001 {
                  tunnel: w5002 -> [w5008 _]
                  tunnel: w5000 -> [w5007 _]
                  tunnel: w4999 -> [w5006 _]
                  frame False {
                    n1842 = case shown="True" w5008 {
                      frame False {
                        n1843 = local write "Y1 2"(TRUE ("X1 4")) -> ()
                        n1844 = local write "Y 2"(FALSE ("X 4")) -> ()
                      }
                      frame True {
                        n1845 = local write "error"(TRUE ("X1 4")) -> ()
                        n1846 = local write "Y 2"(FALSE ("X 4")) -> ()
                      }
                    }
                    n1847 = local write "10R Y(k-1)"(w5006) -> ()
                    n1848 = local write "input 2 y [10R]"(w5006) -> ()
                    n1849 = local write "output 1 y [10R]"(w5007) -> ()
                  }
                  frame True {
                  }
                }
              }
            }
            n1850 = case shown="True" "X1 2" {
              frame False {
              }
              frame True {
                n1851 = local read "İterasyon X 2"() -> (w5076:dbl)
                n1852 = local read "output 1 x [10R]"() -> (w5079:dbl)
                n1853 = local read "10R X(k-1)"() -> (w5078:dbl)
                n1854 = local read "10R Xk"() -> (w5077:dbl)
                n1855 = call "X1.vi"("denge degeri"=2.0, "İterasyon Denge"=w5076, "Xk"=w5077, "X(k-1)"=w5078, "output x 1"=w5079) -> ("Output Xk"=w5072:dbl, "output x 2"=w5071:dbl, "cycle"=w5073:bool, "error"=w5074:bool)  [unwired: 7 in]
                n1856 = case shown="False" w5073 {
                  tunnel: w5074 -> [w5082 _]
                  tunnel: w5072 -> [w5081 _]
                  tunnel: w5071 -> [w5080 _]
                  frame False {
                    n1857 = case shown="True" w5082 {
                      frame False {
                        n1858 = local write "RANGE KONTROL X 2"(TRUE ("RANGE KONTROL X 4")) -> ()
                        n1859 = local write "X1 2"(FALSE ("X1 4")) -> ()
                      }
                      frame True {
                        n1860 = local write "X1 2"(FALSE ("X1 4")) -> ()
                        n1861 = local write "error"(TRUE ("X1 4")) -> ()
                      }
                    }
                    n1862 = local write "10R Xk"(w5081) -> ()
                    n1863 = local write "output 2 x [10R]"(w5080) -> ()
                  }
                  frame True {
                  }
                }
              }
            }
            n1864 = case shown="True" "Y1 2" {
              frame False {
              }
              frame True {
                n1865 = local read "İterasyon Y 2"() -> (w4988:dbl)
                n1866 = local read "output 1 y [10R]"() -> (w4991:dbl)
                n1867 = local read "10R Y(k-1)"() -> (w4990:dbl)
                n1868 = local read "10R Yk"() -> (w4989:dbl)
                n1869 = call "Y1.vi"("denge degeri"=2.0, "İterasyon Denge"=w4988, "Yk"=w4989, "Y(k-1)"=w4990, "output y 1"=w4991) -> ("Output Yk"=w4984:dbl, "output y 2"=w4983:dbl, "cycle"=w4985:bool, "error"=w4986:bool)  [unwired: 7 in]
                n1870 = case shown="False" w4985 {
                  tunnel: w4986 -> [w4994 _]
                  tunnel: w4984 -> [w4993 _]
                  tunnel: w4983 -> [w4992 _]
                  frame False {
                    n1871 = case shown="False" w4994 {
                      frame False {
                        n1872 = local write "RANGE KONTROL Y 2"(TRUE ("RANGE KONTROL X 4")) -> ()
                        n1873 = local write "Y1 2"(FALSE ("X1 4")) -> ()
